vi "Histogram Main.vi"() -> ()   [LabVIEW 2015]
uses:
  Consumer Message.ctl
  <vilib>/Utility/file.llb/Write Delimited Spreadsheet (DBL).vi
  <vilib>/ErrorRing/Error Ring.xnode
panel:
  in  "bins":i32=20
  out "Histogram":cluster{"histogram":dbl[], "x axis":dbl[]}(graph)
  in  "signal":u16(ring) items=["uniform white", "uniform+uniform", "Gaussian white", "sine", "square"]
  out "Consumer Shutdown?":bool
  out "State to Execute":string
  out "Backlog":u8(slide) scale=0.0..100.0
  in  "Snapshot":bool
  in  "Stop":bool
  # "Number of enqueued messages waiting to be processed"
  # "Current data being processed in consumer loop"
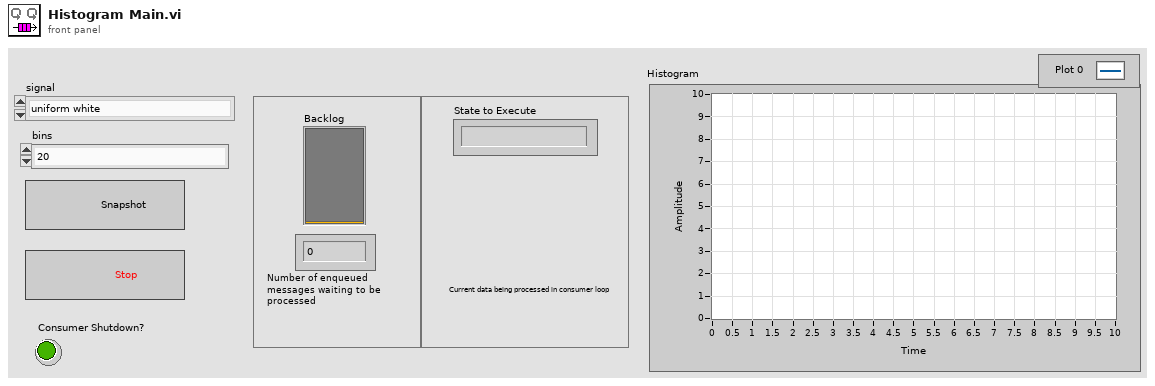
[diagram p1: front panel]
types:
  T1 = typedef "Consumer Message.ctl" = cluster{"Consumer State":string, "Boolean Data":bool, "Numeric Data":i32, "Signal":dbl[], "Error":errorcluster}
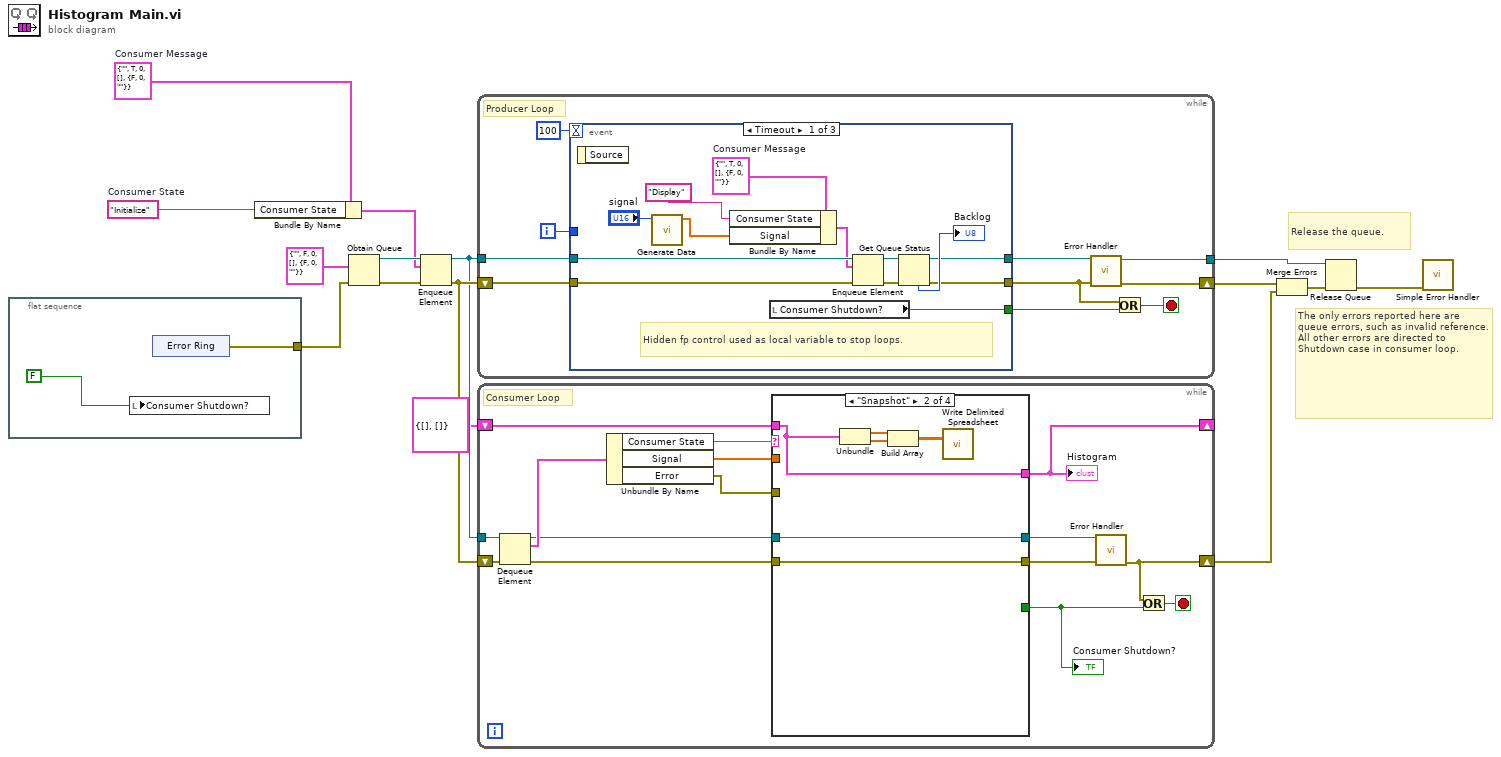
[diagram p0: block diagram]
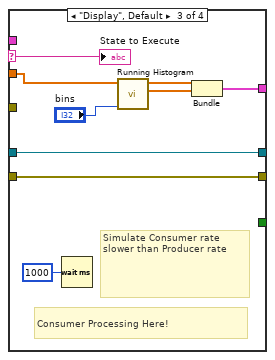
[diagram p3: hidden frame]
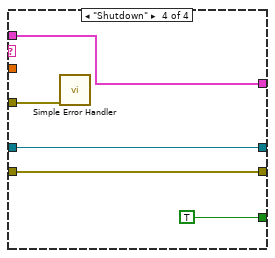
[diagram p4: hidden frame]
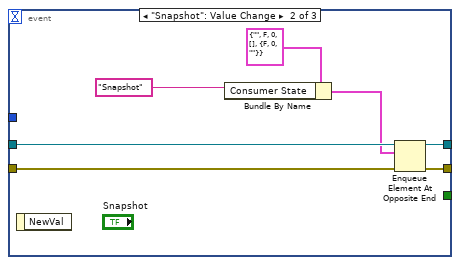
[diagram p5: hidden frame]
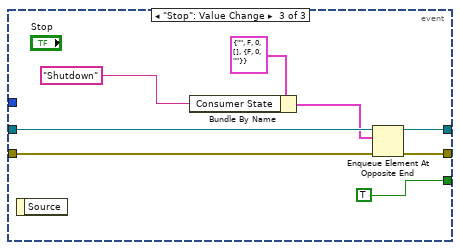
[diagram p6: hidden frame]
diagram:
  w7 = "Initialize"  # Consumer State
  w9 = T1 {"Consumer State"="", "Boolean Data"=TRUE, "Numeric Data"=0, "Signal"=[], "Error"={"status"=FALSE, "code"=0, "source"=""}}  # Consumer Message
  # "Release the queue."
  # "The only errors reported here are queue errors, such as invalid reference.  All other errors are directed to Shutdown case in consumer loop."
  n1 = flat-sequence {
    tunnel: [w16] -> w10
    frame #0 {
      n2 = local write "Consumer Shutdown?"(FALSE ("Stop Loops (local)")) -> ()
      n3 = xnode "Error Ring"() -> ("error out"=w16:errorcluster)
    }
  }
  n4 = Bundle By Name(cluster=w9, "Consumer State"=w7) -> (w8:T1)
  n5 = Obtain Queue(element data type=T1 {"Consumer State"="", "Boolean Data"=FALSE, "Numeric Data"=0, "Signal"=[], "Error"={"status"=FALSE, "code"=0, "source"=""}}, error in (no error)=w10) -> (queue out=w12:refnum<queue>, error out=w15:errorcluster)  [unwired: 3 in, 1 out]
  n6 = Enqueue Element(queue=w12, element=w8, error in (no error)=w15) -> (queue out=w11:refnum<queue>, error out=w13:errorcluster)  [unwired: 1 in, 1 out]
  n7 = while {
    tunnel: w11 -> [w28]
    shift-right: [w20] -> w6
    shift-left: w13 -> [w27]
    tunnel: [w19] -> w2
    i -> [w26]
    stop <- w22 stop-if-true
    # "Producer Loop"
    n8 = event shown="[0] Timeout" {
      selector: _ -> [_ _ _]
      dyn-events: _ -> [_ _ _]
      timeout: 100 -> [_ _ _]
      tunnel: w28 -> [w39 w47 w56]
      tunnel: w27 -> [w31 w46 w54]
      tunnel: [w38 w48 w53] -> w21
      tunnel: [w41 _ TRUE] -> w23
      tunnel: w26 -> [_ _ _]
      tunnel: [w37 w43 w52] -> w25
      event Timeout {
        w36 = T1 {"Consumer State"="", "Boolean Data"=TRUE, "Numeric Data"=0, "Signal"=[], "Error"={"status"=FALSE, "code"=0, "source"=""}}  # Consumer Message
        # "Hidden fp control used as local variable to stop loops."
        n9 = event-data() -> ()  [unwired: 1 in, 1 out]
        n10 = call "Generate Data.vi"("signal"="signal") -> ("Y"=w35:dbl[])  [unwired: 9 in, 1 out]
        n11 = Bundle By Name(cluster=w36, "Consumer State"="Display", "Signal"=w35) -> (w29:T1)
        n12 = local read "Consumer Shutdown?"() -> (w41:bool)
        n13 = Enqueue Element(queue=w39, element=w29, error in (no error)=w31) -> (queue out=w32:refnum<queue>, error out=w30:errorcluster)  [unwired: 1 in, 1 out]
        n14 = Get Queue Status(queue=w32, error in (no error)=w30) -> (queue out=w37:refnum<queue>, error out=w38:errorcluster, # elements in queue=→"Backlog":i32)  [unwired: 1 in, 5 out]
      }
      event "Snapshot": Value Change {
        n15 = event-data() -> ()  [unwired: 1 in, 1 out]
        n16 = Bundle By Name(cluster=T1 {"Consumer State"="", "Boolean Data"=FALSE, "Numeric Data"=0, "Signal"=[], "Error"={"status"=FALSE, "code"=0, "source"=""}}, "Consumer State"="Snapshot" ("String Data")) -> (w44:T1)
        n17 = Enqueue Element At Opposite End(queue=w47, element=w44, error in (no error)=w46) -> (queue out=w43:refnum<queue>, error out=w48:errorcluster)  [unwired: 1 in, 1 out]
      }
      event "Stop": Value Change {
        n18 = event-data() -> ()  [unwired: 1 in, 1 out]
        n19 = Bundle By Name(cluster=T1 {"Consumer State"="", "Boolean Data"=FALSE, "Numeric Data"=0, "Signal"=[], "Error"={"status"=FALSE, "code"=0, "source"=""}}, "Consumer State"="Shutdown") -> (w49:T1)
        n20 = Enqueue Element At Opposite End(queue=w56, element=w49, error in (no error)=w54) -> (queue out=w52:refnum<queue>, error out=w53:errorcluster)  [unwired: 1 in, 1 out]
      }
    }
    n21 = call "Error Handler.vi"("error in"=w21, "queue in"=w25) -> ("error out"=w20:errorcluster, "queue out"=w19:refnum<queue>)  [unwired: 8 in]
    n22 = Or(x=w21, y=w23) -> (x .or. y?=w22:bool)
  }
  n23 = while {
    tunnel: w11 -> [w71]
    shift-right: [w62] -> w5
    shift-left: w13 -> [w70]
    shift-right: [w58] -> _
    shift-left: cluster{"histogram":dbl[], "x axis":dbl[]} {"histogram"=[], "x axis"=[]} -> [w57]
    stop <- w63 stop-if-true
    # "Consumer Loop"
    n24 = Dequeue Element(queue=w71, error in (no error)=w70) -> (queue out=w61:refnum<queue>, element=w69:T1, error out=w60:errorcluster)  [unwired: 1 in, 1 out]
    n25 = Unbundle By Name(w69) -> ("Consumer State"=w68:string, "Signal"=w67:dbl[], "Error"=w59:errorcluster)
    n26 = case shown="\"Snapshot\"" w68 {
      selector: w68 -> [_ _ w88 _]
      tunnel: [_ _ _ TRUE] -> w64
      tunnel: w60 -> [w73 w79 w86 w91]
      tunnel: [w73 w79 w86 w91] -> w66
      tunnel: w67 -> [_ _ w85 _]
      tunnel: w61 -> [w74 w80 w89 w92]
      tunnel: [w74 w80 w89 w92] -> w65
      tunnel: w59 -> [_ _ _ w93]
      tunnel: [w72 w78 w81 w90] -> w58
      tunnel: w57 -> [w72 w78 _ w90]
      frame "Initialize" {
      }
      frame "Snapshot" {
        n27 = Unbundle(w78) -> ("histogram"=w77:dbl[], "x axis"=w76:dbl[])
        n28 = Build Array(w77, w76) -> (w75:dbl[][])
        n29 = call-poly <vilib>:"Write Delimited Spreadsheet.vi"("2D data"=w75) -> ()  [unwired: 13 in, 2 out]
      }
      frame "Display", Default {
        # "Simulate Consumer rate slower than Producer rate"
        # "Consumer Processing Here!"
        n30 = Wait (ms)(milliseconds to wait=u32 1000) -> ()  [unwired: 1 out]
        n31 = call "Running Histogram.vi"("bins"="bins", "input data"=w85) -> ("x axis"=w82:dbl[], "histogram"=w83:dbl[])  [unwired: 6 in, 2 out]
        n32 = Bundle("histogram"=w83, "x axis"=w82) -> (w81:cluster{"histogram":dbl[], "x axis":dbl[]})  [unwired: 1 in]
        "State to Execute" <- w88
      }
      frame "Shutdown" {
        n33 = call <vilib>:"Simple Error Handler.vi"("error in (no error)"=w93) -> ()  [unwired: 4 in, 5 out]
      }
    }
    "Consumer Shutdown?" <- w64
    "Histogram" <- w58
    n34 = call "Error Handler.vi"("error in"=w66, "queue in"=w65) -> ("error out"=w62:errorcluster)  [unwired: 8 in, 1 out]
    n35 = Or(x=w62, y=w64) -> (x .or. y?=w63:bool)
  }
  n36 = Merge Errors(w6, w5) -> (w4:errorcluster)
  n37 = Release Queue(queue=w2, error in (no error)=w4) -> (error out=w3:errorcluster)  [unwired: 1 in, 2 out]
  n38 = call <vilib>:"Simple Error Handler.vi"("error in (no error)"=w3) -> ()  [unwired: 4 in, 5 out]
